vi "Analog DAQ-Core_Initialize.vi"(0 "Initialization Sequence":string, 5 "FTW Actor Instance Configuration":string, 11 "error in (no error)":errorcluster) -> (4 "Analog DAQ-Core Out":refnum<class "Analog DAQ-Core.lvclass">, 6 "Event Refnums":T1, 15 "error out":errorcluster)   [LabVIEW 2018, in "Analog DAQ-Core.lvclass"]
uses:
  Analog DAQ-Core.lvclass
  source/actor/Message/Request/FTW-Message-IncomingRequest.lvclass
  source/actor/Message/Base/FTW-Message.lvclass
  Analog DAQ-Core.lvclass/Analog DAQ-Core.ctl
  0953a831-09d8-4f24-9d0d-b74cc592a5c0.vi
  source/JSON/core/FTW-JSON-Core-EncodingFlags.vi
  source/Reflection/FTW-Reflection-Type.vi
  source/JSON/FTW-JSON-Parse.vi
  source/container/FTW-Container-GetFlattenedValue.vi
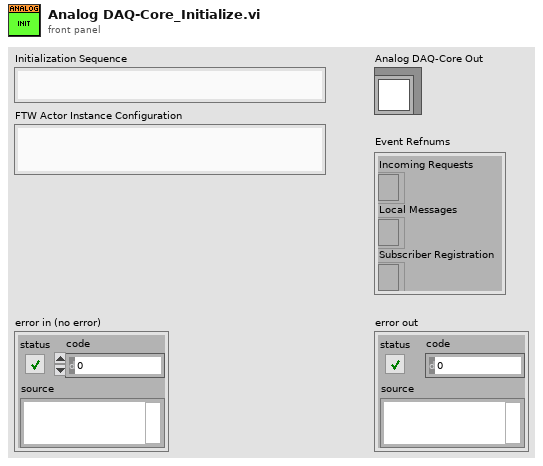
[diagram p1: front panel]
types:
  T1 = cluster{"Incoming Requests":refnum<event-registration>, "Local Messages":refnum<event-registration>, "Subscriber Registration":refnum<event-registration>}
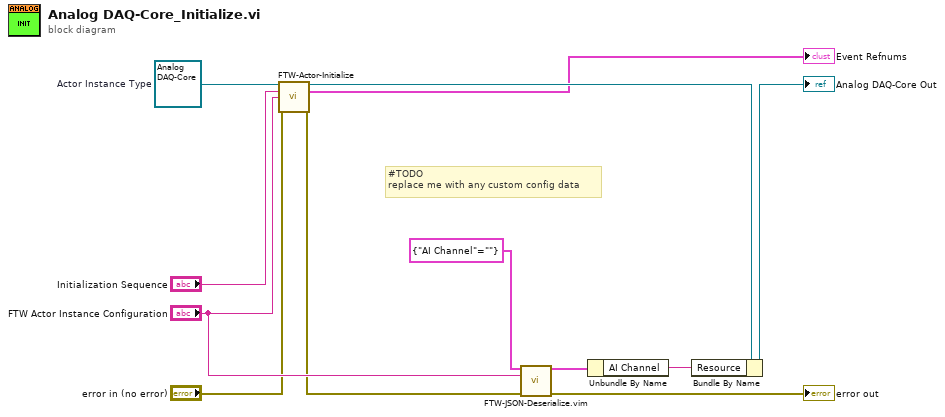
[diagram p0: block diagram]
diagram:
  w4 = refnum<class "Analog DAQ-Core.lvclass"> refnum  # Actor Instance Type
  # "#TODO\nreplace me with any custom config data"
  n1 = call-dynamic "FTW-Actor-Initialize.vi"("FTW Actor Instance Type"=w4, "Initialization Job Sequence"="Initialization Sequence", "Actor Instance Configuration"="FTW Actor Instance Configuration", "error in"="error in (no error)") -> ("FTW Actor Instance"=w3:refnum<class "Analog DAQ-Core.lvclass">, "Event Refnums"=→"Event Refnums":T1, "error out"=w6:errorcluster)  [unwired: 9 in]
  n2 = call "FTW-JSON-Deserialize.vim"("Type In"=cluster{"AI Channel":string} {"AI Channel"=""} ("Type and Defaults"), "JSON String"="FTW Actor Instance Configuration", "error in"=w6) -> ("Type Out"=w9:cluster{"AI Channel":string}, "error out"=→"error out":errorcluster)  [unwired: 11 in]
  n3 = Unbundle By Name(w9) -> ("AI Channel"=w8:string)
  n4 = Bundle By Name(cluster=w3, "Resource"=w8) -> (→"Analog DAQ-Core Out":refnum<class "Analog DAQ-Core.lvclass">)
